vi "LabviewMusicPlayer.vi"() -> ()   [LabVIEW 2021]
uses:
  <vilib>/sound2/lvsound2.llb/Sampling Mode.ctl
  <vilib>/sound2/lvsound2.llb/Sound File Position.ctl
  <vilib>/sound2/lvsound2.llb/Sound File Read Open.vi
  <vilib>/sound2/lvsound2.llb/Sound File Info (refnum).vi
  <vilib>/sound2/lvsound2.llb/Sound File Read (DBL).vi
  <vilib>/measure/maspectr.llb/FFT Spectrum (Mag-Phase) for N Chan.vi
  <vilib>/sound2/lvsound2.llb/Sound Output Write (DBL).vi
  <vilib>/measure/NI_MAPro.lvlib
panel:
  out "Numeric 2":dbl format="%#.1g"
  out "Numeric":dbl
  out "Lista":string
  in  "next L":bool
  out "Lista":string[](array[string])
  in  "Retroceder":bool
  in  "Avanzar":bool
  in  "Pause":bool
  in  "Stop":bool
  in  "Play":bool
  in  "prev c":bool
  in  "next c":bool
  out "Artista":string
  out "Canción":string
  out "?":sgl(slide) scale=0.0..1.0 scale format="%.6g"
  in  "stop 2":bool
  in  "prev L":bool
  out "Frecuencia":cluster{"f0":dbl, "df":dbl, "magnitude":dbl[]}[](graph)
  out "Tiempo":waveform(dbl)[](graph)
  in  "Path":path
  # "Canciones"
  # "M"
  # "S"
  # "Hernandez Orozco Cesar Gibran 3MV7 Instrumentacion Virtual 2024-2"
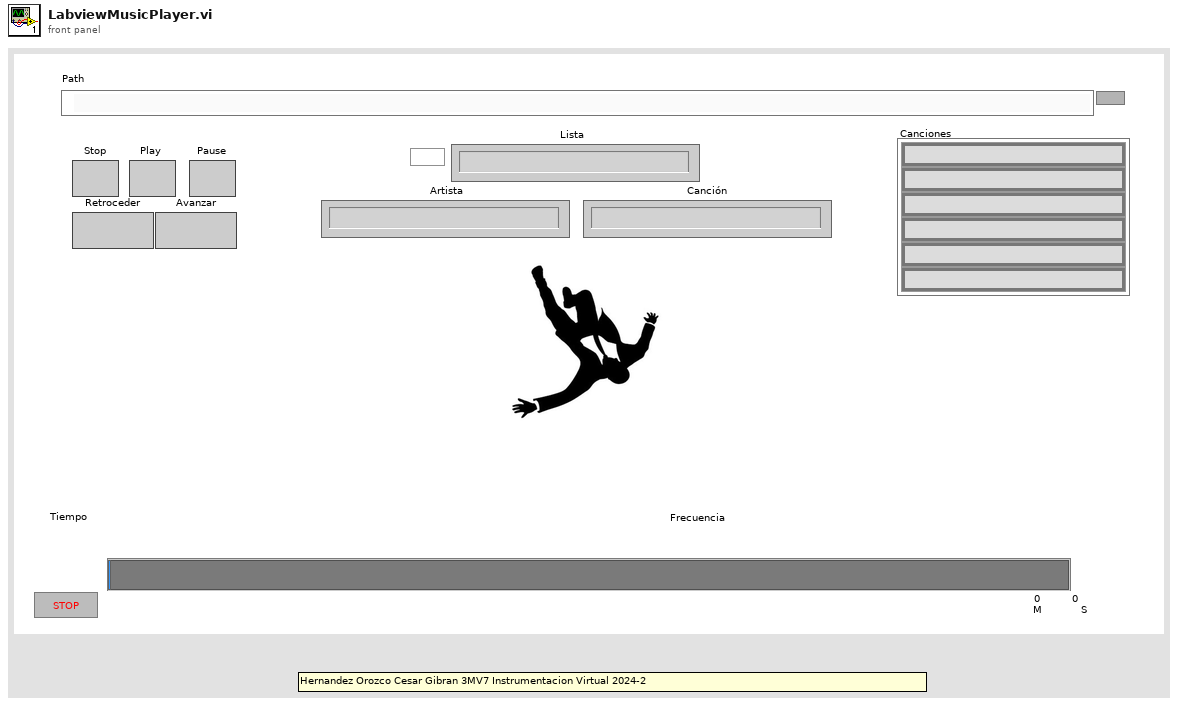
[diagram p1: front panel]
types:
  T1 = typedef "Sampling Mode.ctl" = i32
  T2 = typedef "Sound File Refnum.ctl" = refnum<file>
  T3 = typedef "Sound Data Format.ctl" = cluster{"sample rate (S/s)":dbl, "number of channels":i32, "bits per sample":i32}
  T4 = typedef "Sound Output Task ID.ctl" = u32
  T5 = typedef "Sound File Position.ctl" = u16
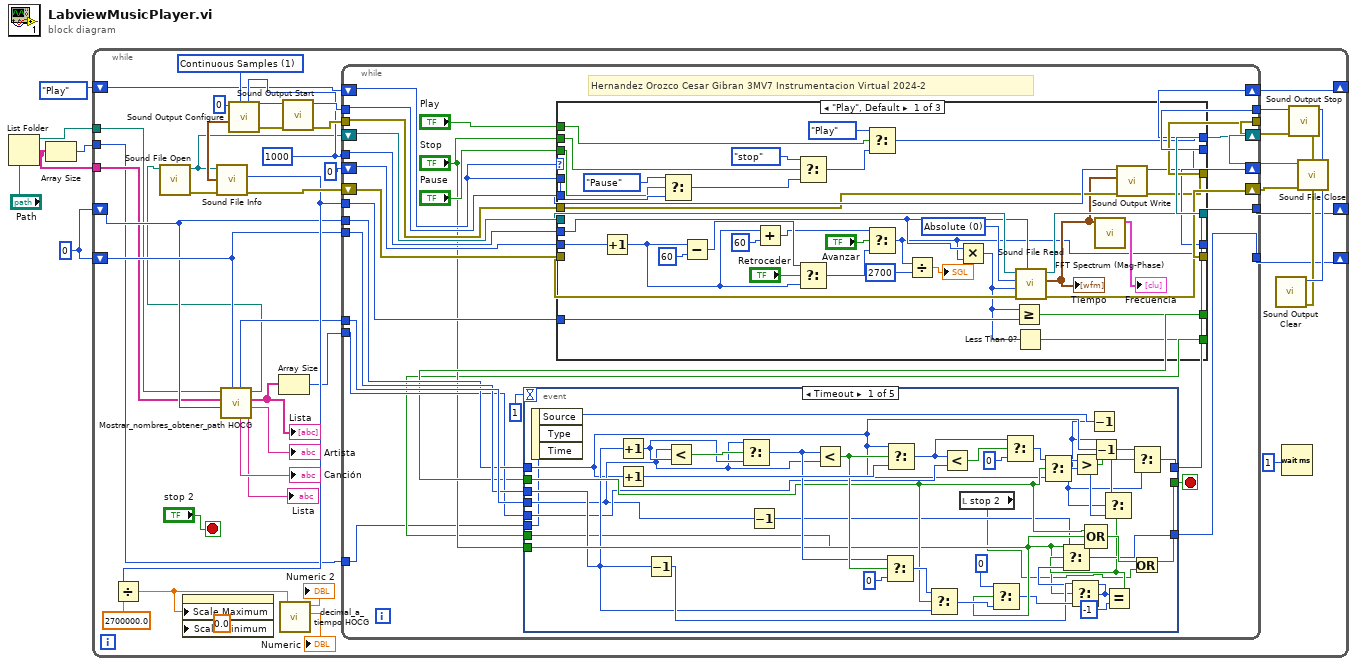
[diagram p0: block diagram]
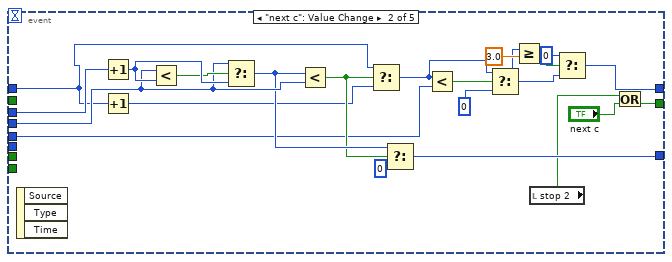
[diagram p2: hidden frame]
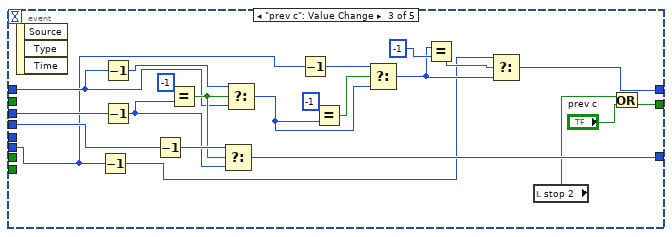
[diagram p3: hidden frame]
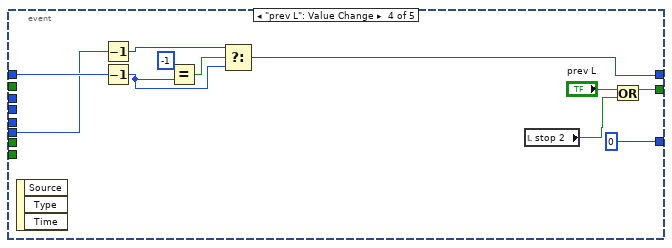
[diagram p4: hidden frame]
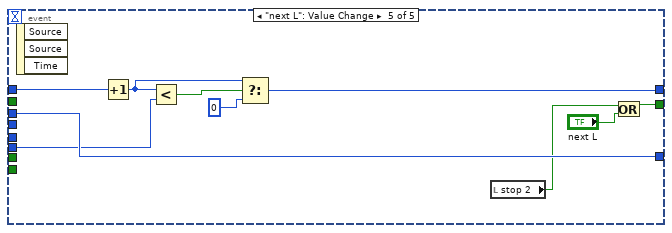
[diagram p5: hidden frame]
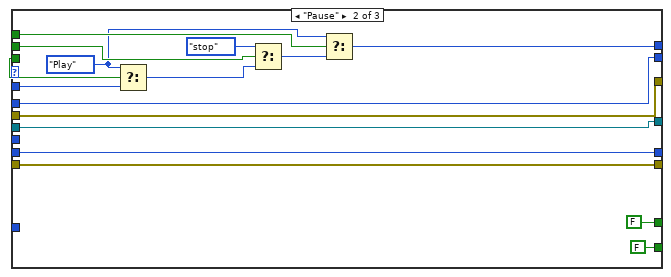
[diagram p6: hidden frame]
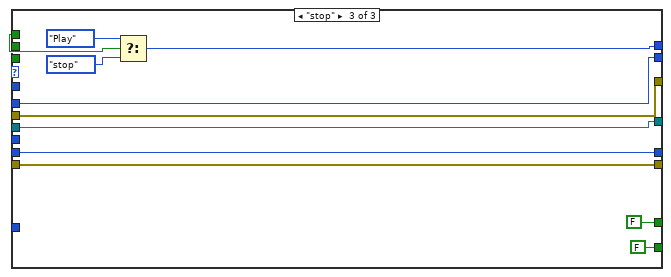
[diagram p7: hidden frame]
diagram:
  w1 = 0
  n1 = List Folder(path="Path") -> (path out=w5:path, folder names=w3:string[])  [unwired: 3 in, 2 out]
  n2 = Array Size(array=w3) -> (size(s)=w2:i32)
  n3 = while {
    shift-right: [w27] -> _
    shift-left: w1 -> [w20]
    tunnel: w3 -> [w14]
    tunnel: w5 -> [w13]
    shift-right: [w26] -> _
    shift-left: w1 -> [w21]
    shift-right: [w30] -> _
    shift-left: enum16{"Play", "Pause", "stop"}."Play" ("Listas de reproducción") -> [w19]
    tunnel: w2 -> [w11]
    stop <- "stop 2" stop-if-true
    w24 = 1000 ("number of samples/ch")
    w35 = T1 1 items=["Finite Samples", "Continuous Samples"] ("sample mode")
    n4 = call "Mostrar_nombres_obtener_path HOCG.vi"("Cancion actual"=w21, "Lista actual"=w20, "folder names"=w14, "path in"=w13) -> ("Lista actual"=→"Lista":string, "Artista"=→"Artista":string, "Lista"=w15:string[], "Path de cancion"=w12:path, "Canción"=→"Canción":string, "Cantidad de canciones"=w29:i32)  [unwired: 2 in]
    "Lista" <- w15
    n5 = call-poly <vilib>:"Sound File Open.vi"("path"=w12) -> ("error out"=w23:errorcluster, "sound file refnum"=w22:T2)  [unwired: 9 in]
    n6 = call-poly <vilib>:"Sound File Info.vi"("error in (no error)"=w23, "sound file refnum"=w22) -> ("error out"=w43:errorcluster, "sound format"=w36:T3, "total number of samples/ch"=w31:u32)  [unwired: 6 in, 1 out]
    n7 = Divide(x=w31, y=2700000.0) -> (x/y=w9:dbl)
    n8 = property class="Slide (strict)"("Scale.Maximum"=w9, "Scale.Minimum"=0.0 ("Scale.Range:Minimum")) -> ()  [unwired: 2 in, 2 out]
    n9 = call <vilib>:"Sound Output Configure.vi"("number of samples/ch"=w24, "sample mode"=w35, "sound format"=w36, "device ID"=u32 0) -> ("error out"=w37:errorcluster, "task ID"=w38:T4)  [unwired: 6 in]
    n10 = Array Size(array=w15) -> (size(s)=w28:i32)
    n11 = call "decimal_a_tiempo HOCG.vi"("Numeric 3"=w9) -> ("Numeric"=→"Numeric":dbl, "Numeric 2"=→"Numeric 2":dbl)  [unwired: 9 in]
    n12 = call <vilib>:"Sound Output Start.vi"("error in (no error)"=w37, "task ID"=w38) -> ("error out"=w44:errorcluster, "task ID out"=w45:T4)  [unwired: 8 in]
    n13 = while {
      tunnel: w45 -> [w76]
      tunnel: w44 -> [w75]
      tunnel: w24 -> [w72]
      shift-right: [w71] -> w42
      shift-left: w22 -> [w74]
      shift-right: [w70] -> w41
      shift-left: w43 -> [w73]
      tunnel: [w69] -> w10
      tunnel: [w68] -> w40
      shift-right: [w64] -> w30
      shift-left: w19 -> [w65]
      shift-right: [w66] -> _
      shift-left: 0 ("number of samples/ch") -> [w67]
      tunnel: w31 -> [w61]
      tunnel: w29 -> [w60]
      tunnel: w21 -> [w59]
      tunnel: w20 -> [w58]
      tunnel: w28 -> [w57]
      tunnel: [w56] -> w27
      tunnel: [w55] -> w26
      tunnel: w11 -> [w49]
      stop <- w52 stop-if-true
      # "Hernandez Orozco Cesar Gibran 3MV7 Instrumentacion Virtual 2024-2"
      n14 = case shown="\"Play\", Default" w65 {
        tunnel: w76 -> [w216 w231 w240]
        tunnel: w75 -> [w215 w232 w239]
        tunnel: w74 -> [w214 w229 w242]
        tunnel: w73 -> [w213 w230 w241]
        tunnel: w72 -> [w194 _ _]
        tunnel: [w211 w229 w242] -> w71
        tunnel: [w210 w230 w241] -> w70
        tunnel: [w209 w231 w240] -> w69
        tunnel: [w208 w232 w239] -> w68
        tunnel: w67 -> [w205 w228 w243]
        tunnel: [w180 w228 w243] -> w66
        tunnel: w65 -> [w202 w225 _]
        tunnel: [w195 w219 w234] -> w64
        tunnel: "Pause" -> [w200 w226 _]
        tunnel: "Stop" -> [w199 w223 _]
        tunnel: "Play" -> [w198 w222 w237]
        tunnel: w61 -> [w185 _ _]
        tunnel: [w184 FALSE FALSE] -> w53
        tunnel: [w182 FALSE FALSE] -> w50
        frame "Play", Default {
          w212 = T5 0 items=["Absolute"=0, "Relative"=2] ("position mode")
          n15 = Increment(x=w205) -> (x+1=w189:i32)
          n16 = Select(t=enum16{"Play", "Pause", "stop"}."Pause" ("Listas de reproducción"), s=w200, f=w202) -> (s? t:f=w201:enum16{"Play", "Pause", "stop"})
          n17 = Subtract(x=w189, y=60) -> (x-y=w193:i32)
          n18 = Add(x=w189, y=60) -> (x+y=w187:i32)
          n19 = Select(t=enum16{"Play", "Pause", "stop"}."stop" ("Listas de reproducción"), s=w199, f=w201) -> (s? t:f=w196:enum16{"Play", "Pause", "stop"})
          n20 = Select(t=w193, s="Retroceder", f=w189) -> (s? t:f=w186:i32)
          n21 = Select(t=enum16{"Play", "Pause", "stop"}."Play" ("Listas de reproducción"), s=w198, f=w196) -> (s? t:f=w195:enum16{"Play", "Pause", "stop"})
          n22 = Select(t=w187, s="Avanzar", f=w186) -> (s? t:f=w180:i32)
          n23 = Divide(x=w180, y=2700) -> (x/y=→"?":dbl)
          n24 = Multiply(x=w194, y=w180) -> (x*y=w183:i32)
          n25 = Greater Or Equal?(x=w183, y=w185) -> (x >= y?=w184:bool)
          n26 = Less Than 0?(x=w183) -> (x < 0?=w182:bool)
          n27 = call-poly <vilib>:"Sound File Read.vi"("number of samples/ch (-1: all)"=w194, "error in (no error)"=w213, "position offset"=w183, "position mode"=w212, "sound file refnum"=w214) -> ("error out"=w210:errorcluster, "data"=w207:waveform(dbl)[], "sound file refnum out"=w211:T2)  [unwired: 2 in, 2 out]
          "Tiempo" <- w207
          n28 = call-poly <vilib>:"FFT Spectrum (Mag-Phase).vi"("time signals"=w207) -> ("magnitudes"=→"Frecuencia":cluster{"f0":dbl, "df":dbl, "magnitude":dbl[]}[])  [unwired: 6 in, 4 out]
          n29 = call-poly <vilib>:"Sound Output Write.vi"("error in (no error)"=w215, "data"=w207, "task ID"=w216) -> ("error out"=w208:errorcluster, "task ID out"=w209:T4)  [unwired: 7 in]
        }
        frame "Pause" {
          w221 = enum16{"Play", "Pause", "stop"}."Play" ("Listas de reproducción")
          n30 = Select(t=w221, s=w226, f=w225) -> (s? t:f=w224:enum16{"Play", "Pause", "stop"})
          n31 = Select(t=enum16{"Play", "Pause", "stop"}."stop" ("Listas de reproducción"), s=w223, f=w224) -> (s? t:f=w220:enum16{"Play", "Pause", "stop"})
          n32 = Select(t=w221, s=w222, f=w220) -> (s? t:f=w219:enum16{"Play", "Pause", "stop"})
        }
        frame "stop" {
          n33 = Select(t=enum16{"Play", "Pause", "stop"}."Play" ("Listas de reproducción"), s=w237, f=enum16{"Play", "Pause", "stop"}."stop" ("Listas de reproducción")) -> (s? t:f=w234:enum16{"Play", "Pause", "stop"})
        }
      }
      n34 = event shown="[0] Timeout" {
        selector: _ -> [_ _ _ _ _]
        dyn-events: _ -> [_ _ _ _ _]
        timeout: 1 -> [_ _ _ _ _]
        tunnel: w60 -> [w86 w132 w154 _ _]
        tunnel: w59 -> [w95 w135 w156 _ w173]
        tunnel: w58 -> [w85 w121 w148 w165 w175]
        tunnel: [w78 w115 w137 w159 w170] -> w52
        tunnel: w57 -> [w87 w126 _ _ _]
        tunnel: [w82 w116 w143 w163 w171] -> w56
        tunnel: [w91 w123 w150 u32 0 ("f") w173] -> w55
        tunnel: w53 -> [w99 _ _ _ _]
        tunnel: "Stop" -> [w98 _ _ _ _]
        tunnel: w50 -> [w80 _ _ _ _]
        tunnel: w49 -> [w81 _ w138 w160 w172]
        event Timeout {
          n35 = event-data() -> ()  [unwired: 1 in, 3 out]
          n36 = Increment(x=w95) -> (x+1=w109:u32)
          n37 = Increment(x=w85) -> (x+1=w111:u32)
          n38 = Decrement(x=w95) -> (x-1=w96:u32)
          n39 = Less?(x=w86, y=w109) -> (x < y?=w110:bool)
          n40 = Select(t=w86, s=w110, f=w109) -> (s? t:f=w103:u32)
          n41 = Decrement(x=w86) -> (x-1=w92:i32)
          n42 = Less?(x=w103, y=w86) -> (x < y?=w106:bool)
          n43 = Select(t=w103, s=w106, f=u32 0) -> (s? t:f=w105:u32)
          n44 = Select(t=w85, s=w106, f=w111) -> (s? t:f=w113:u32)
          n45 = Select(t=w105, s=w99, f=w95) -> (s? t:f=w101:u32)
          n46 = Less?(x=w113, y=w87) -> (x < y?=w112:bool)
          n47 = local read "stop 2"() -> (w77:bool)
          n48 = Select(t=u32 0, s=w98, f=w101) -> (s? t:f=w97:u32)
          n49 = Select(t=w113, s=w112, f=u32 0) -> (s? t:f=w104:u32)
          n50 = Select(t=w104, s=w99, f=w85) -> (s? t:f=w89:u32)
          n51 = Select(t=w96, s=w80, f=w97) -> (s? t:f=w93:u32)
          n52 = Compound Arithmetic op=OR(w99, w98, w80) -> (w100:bool)
          n53 = Decrement(x=w81) -> (x-1=w79:i32)
          n54 = Decrement(x=w85) -> (x-1=w88:u32)
          n55 = Equal?(x=w93, y=-1) -> (x = y?=w90:bool)
          n56 = Select(t=w92, s=w90, f=w93) -> (s? t:f=w91:u32)
          n57 = Select(t=w88, s=w90, f=w89) -> (s? t:f=w83:u32)
          n58 = Greater?(x=w83, y=w79) -> (0:w84:bool)
          n59 = Select(t=w79, s=w84, f=w83) -> (s? t:f=w82:u32)
          n60 = Or(x=w100, y=w77) -> (x .or. y?=w78:bool)
        }
        event "next c": Value Change {
          n61 = event-data() -> ()  [unwired: 1 in, 3 out]
          n62 = Increment(x=w135) -> (x+1=w134:u32)
          n63 = Increment(x=w121) -> (x+1=w127:u32)
          n64 = Less?(x=w132, y=w134) -> (x < y?=w133:bool)
          n65 = Select(t=w132, s=w133, f=w134) -> (s? t:f=w131:u32)
          n66 = Less?(x=w131, y=w132) -> (x < y?=w129:bool)
          n67 = Select(t=w121, s=w129, f=w127) -> (s? t:f=w122:u32)
          n68 = Select(t=w131, s=w129, f=u32 0) -> (s? t:f=w123:u32)
          n69 = Less?(x=w122, y=w126) -> (x < y?=w125:bool)
          n70 = Select(t=w122, s=w125, f=u32 0) -> (s? t:f=w118:u32)
          n71 = Greater Or Equal?(x=w118, y=3.0) -> (x >= y?=w120:bool)
          n72 = local read "stop 2"() -> (w114:bool)
          n73 = Select(t=u32 0, s=w120, f=w118) -> (s? t:f=w116:u32)
          n74 = Or(x=w114, y="next c") -> (x .or. y?=w115:bool)
        }
        event "prev c": Value Change {
          n75 = event-data() -> ()  [unwired: 1 in, 3 out]
          n76 = Decrement(x=w138) -> (x-1=w139:i32)
          n77 = Decrement(x=w148) -> (x-1=w149:u32)
          n78 = Decrement(x=w156) -> (x-1=w152:u32)
          n79 = Decrement(x=w154) -> (x-1=w155:i32)
          n80 = Equal?(x=-1, y=w152) -> (x = y?=w151:bool)
          n81 = Select(t=w155, s=w151, f=w152) -> (s? t:f=w150:u32)
          n82 = Select(t=w149, s=w151, f=w148) -> (s? t:f=w144:u32)
          n83 = Decrement(x=w138) -> (x-1=w145:i32)
          n84 = Equal?(x=-1, y=w144) -> (x = y?=w146:bool)
          n85 = Select(t=w145, s=w146, f=w144) -> (s? t:f=w140:u32)
          n86 = Equal?(x=w140, y=-1) -> (x = y?=w141:bool)
          n87 = Select(t=w139, s=w141, f=w140) -> (s? t:f=w143:u32)
          n88 = local read "stop 2"() -> (w136:bool)
          n89 = Or(x=w136, y="prev c") -> (x .or. y?=w137:bool)
        }
        event "prev L": Value Change {
          n90 = event-data() -> ()  [unwired: 1 in, 3 out]
          n91 = Decrement(x=w160) -> (x-1=w164:i32)
          n92 = Decrement(x=w165) -> (x-1=w166:u32)
          n93 = Equal?(x=-1, y=w166) -> (x = y?=w167:bool)
          n94 = Select(t=w164, s=w167, f=w166) -> (s? t:f=w163:u32)
          n95 = local read "stop 2"() -> (w158:bool)
          n96 = Or(x="prev L", y=w158) -> (x .or. y?=w159:bool)
        }
        event "next L": Value Change {
          n97 = event-data() -> ()  [unwired: 1 in, 3 out]
          n98 = Increment(x=w175) -> (x+1=w174:u32)
          n99 = Less?(x=w174, y=w172) -> (x < y?=w177:bool)
          n100 = Select(t=w174, s=w177, f=u32 0) -> (s? t:f=w171:u32)
          n101 = local read "stop 2"() -> (w169:bool)
          n102 = Or(x=w169, y="next L") -> (x .or. y?=w170:bool)
        }
      }
    }
    n103 = Wait (ms)(milliseconds to wait=u32 1) -> ()  [unwired: 1 out]
    n104 = call <vilib>:"Sound Output Stop.vi"("error in (no error)"=w40, "task ID"=w10) -> ("error out"=w46:errorcluster, "task ID out"=w47:T4)  [unwired: 8 in]
    n105 = call <vilib>:"Sound Output Clear.vi"("error in (no error)"=w46, "task ID"=w47) -> ()  [unwired: 9 in, 1 out]
    n106 = call <vilib>:"Sound File Close.vi"("error in (no error)"=w41, "sound file refnum"=w42) -> ()  [unwired: 9 in, 1 out]
  }
